vi "Set ObjFlags.vi"(8 "error in":errorcluster, 10 "Value":refnum<class "Value.lvclass">, 11 "Object Type in":refnum<class "Object Type Base.lvclass">) -> (0 "error out":errorcluster, 3 "Object Type out":refnum<class "Object Type Base.lvclass">)   [LabVIEW 2024, in "Electronic Datasheet.lvlib" / "Object Type Base.lvclass"]
uses:
  Object Type Base.lvclass
  Value/Value.lvclass
  Object Type Base.lvclass/Object Type Base.ctl
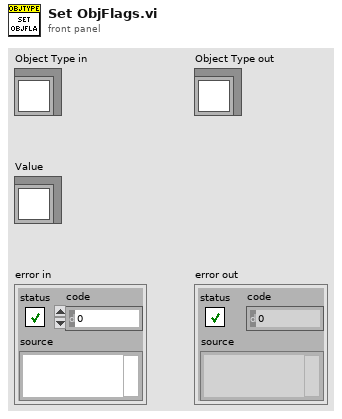
[diagram p1: front panel]
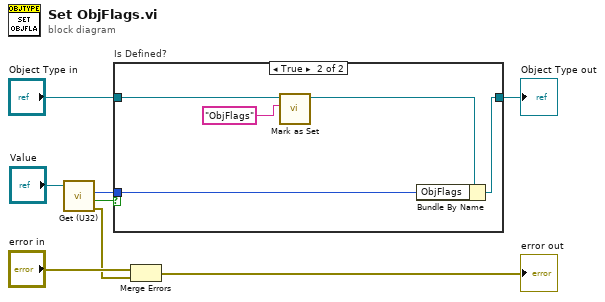
[diagram p0: block diagram]
diagram:
  n1 = call "Get (U32).vi"("Value in"="Value") -> ("error out"=w1:errorcluster, "Is Defined?"=w4:bool, "Value"=w5:u32)  [unwired: 7 in, 1 out]
  n2 = case "Is Defined?" shown="True" w4 {
    tunnel: [w9 w13] -> w7
    tunnel: "Object Type in" -> [w9 w14]
    tunnel: w5 -> [_ w12]
    frame False {
    }
    frame True {
      n3 = call "Mark as Set.vi"("Field name"="ObjFlags", "Object Type in"=w14) -> ("Object Type out"=w11:refnum<class "Object Type Base.lvclass">)  [unwired: 9 in]
      n4 = Bundle By Name(cluster=w11, "ObjFlags"=w12) -> (w13:refnum<class "Object Type Base.lvclass">)
    }
  }
  "Object Type out" <- w7
  n5 = Merge Errors("error in", w1) -> (→"error out":errorcluster)
